vi "Subscribing Groups.vi"(8 "error in (no error)":errorcluster, 11 "LocalGraphBuffer in":refnum<class "LocalGraphBuffer.lvclass">) -> (0 "error out":errorcluster, 2 "Subscribing Groups":string[](array[string]))   [LabVIEW 2020, in "VolatusGUIElements.lvlib" / "LocalGraphBuffer.lvclass"]
uses:
  LocalGraphBuffer.lvclass
  LocalGraphBuffer.lvclass/LocalGraphBuffer.ctl
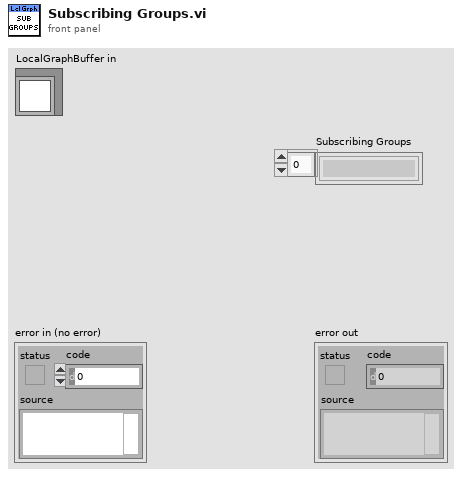
[diagram p1: front panel]
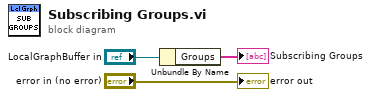
[diagram p0: block diagram]
diagram:
  n1 = Unbundle By Name("LocalGraphBuffer in") -> ("Groups"=→"Subscribing Groups":string[])
  "error out" <- "error in (no error)"
